vi "M11 Power2X.vi"(11 "NXT/EV3":T1) -> (3 "EV3 out":T1)   [LabVIEW 2016]
uses:
  <vilib>/NXT/Subs/LVHSConnector.ctl
  <vilib>/NXT/LegoClasses/BrickReference/BrickReference.lvclass
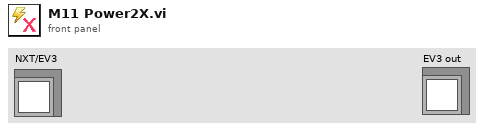
[diagram p1: front panel]
types:
  T1 = typedef "LVHSConnector.ctl" = refnum<class "BrickReference.lvclass">
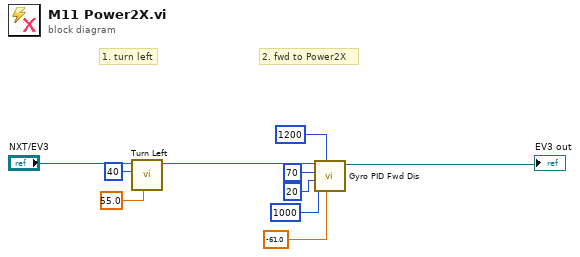
[diagram p0: block diagram]
diagram:
  # "1. turn left"
  # "2. fwd to Power2X"
  n1 = call "Turn Left.vi"("Turning angle"=sgl 55.0, "Motor B (right)"=i8 40, "EV3 in"="NXT/EV3") -> ("EV3 out"=w3:T1)  [unwired: 8 in]
  n2 = call "Gyro PID Fwd Dis.vi"("Target angle"=sgl -61.0, "Threshold to stop"=1200, "Threshold to slow"=1000, "Min. speed"=20, "Max. speed"=70, "EV3 in"=w3) -> ("EV3 out"=→"EV3 out":T1)  [unwired: 5 in]
